vi "GT Set Compensate2D.vi"(8 "error in (no error)":errorcluster caption="错误输入（无错误）", 9 "pComp2d":T1, 10 "axis":i16, 11 "cardNum":i16) -> (0 "error out":errorcluster caption="错误输出", 1 "pComp2d out":T1, 3 "function return":i16)   [LabVIEW 2014, in "gts.lvlib"]
doc: "GT_API GT_SetCompensate2D(short cardNum,short axis,TCompensate2D *pComp2d);"
uses:
  gts.lvlib
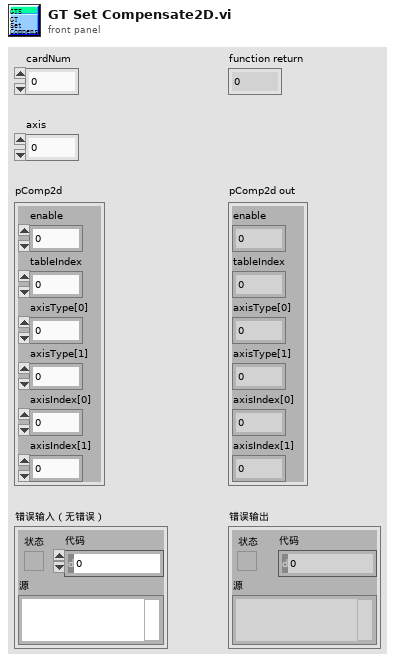
[diagram p1: front panel]
types:
  T1 = cluster{"enable":i16, "tableIndex":i16, "axisType[0]":i16, "axisType[1]":i16, "axisIndex[0]":i16, "axisIndex[1]":i16}
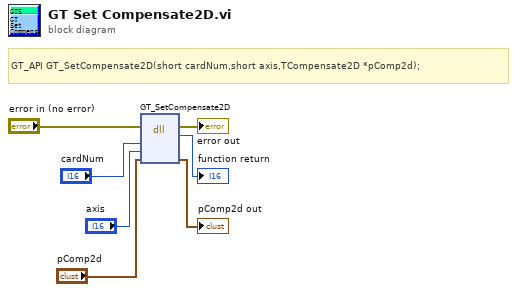
[diagram p0: block diagram]
diagram:
  # "GT_API GT_SetCompensate2D(short cardNum,short axis,TCompensate2D *pComp2d);"
  n1 = dll-call lib="PTH2habs D固高科技资料GTS控制卡GTS卡18年上半年资料dllVC32bit\nmulti_cardgts.*" fn="GT_SetCompensate2D"(error in="error in (no error)", "cardNum"="cardNum", "axis"="axis", "pComp2d"="pComp2d") -> (error out=→"error out":errorcluster, →"function return":i16, "pComp2d"=→"pComp2d out":T1)  [unwired: 4 in, 1 out]
